vi "NT_Array_Names_Test_Code.vi"(8 "Name/Value":string, 10 "Subsystem":T1(ring)) -> ()   [LabVIEW 2019]
panel:
  out "Values":string
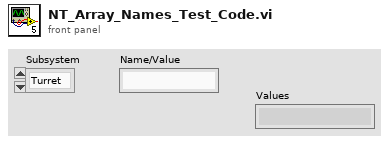
[diagram p1: front panel]
types:
  T1 = enum16{"Turret", "Magazine", "Intake", "Flywheel", "Drive", "Climb"}
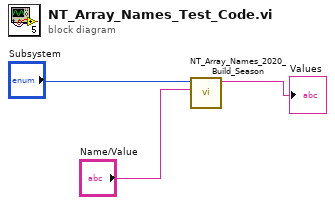
[diagram p0: block diagram]
diagram:
  n1 = call "NT_Array_Names_2020_Build_Season.vi"("Name/Value"="Name/Value", "Subsystem"="Subsystem") -> ("Values"=→"Values":string)  [unwired: 9 in]
